vi "Read Plugin Data.vi"(8 "error in (no error)":errorcluster) -> (0 "error out":errorcluster, 2 "Queue Exists? Yes (T) No (F)":bool, 3 "Plugin Data":refnum<class "Generic Plugin.lvclass">)   [LabVIEW 2011, in "Generic Plugin.lvclass"]
uses:
  Generic Plugin.lvclass
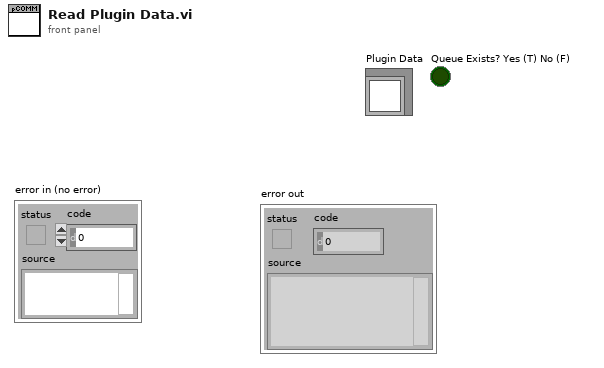
[diagram p1: front panel]
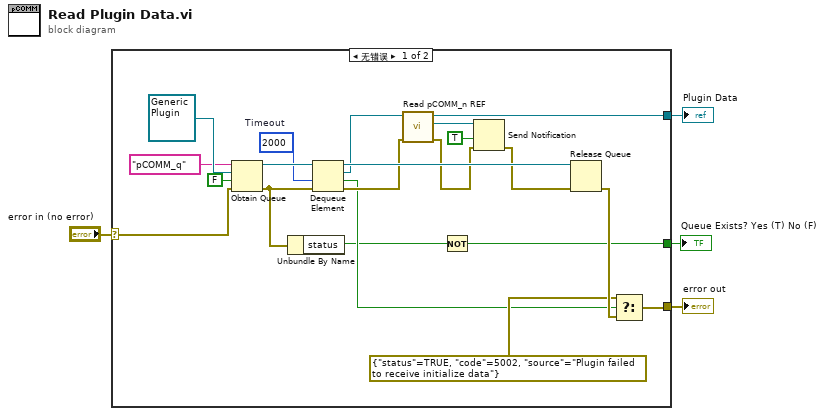
[diagram p0: block diagram]
diagram:
  n1 = case shown="无错误" "error in (no error)" {
    selector: "error in (no error)" -> [w23 w26]
    tunnel: [w18 w26] -> w4
    tunnel: [w14 _] -> w2
    tunnel: [w5 _] -> w1
    frame No Error {
      w21 = 2000  # Timeout
      n2 = Obtain Queue(name (unnamed)="pCOMM_q", element data type=refnum<class "Generic Plugin.lvclass"> refnum ("Generic Plugin.lvclass"), create if not found? (T)=FALSE, error in (no error)=w23) -> (queue out=w22:refnum<queue>, error out=w7:errorcluster)  [unwired: 1 in, 1 out]
      n3 = Unbundle By Name(w7) -> ("status"=w6:bool)
      n4 = Dequeue Element(queue=w22, timeout in ms (-1)=w21, error in (no error)=w7) -> (queue out=w17:refnum<queue>, element=w15:refnum<class "Generic Plugin.lvclass">, timed out?=w8:bool, error out=w11:errorcluster)
      n5 = call "Read pCOMM_n REF.vi"("error in (no error)"=w11, "Generic Plugin in"=w15) -> ("error out"=w10:errorcluster, "pCOMM_n REF"=w13:refnum<notifier>, "Generic Plugin out"=w14:refnum<class "Generic Plugin.lvclass">)  [unwired: 7 in]
      n6 = Not(x=w6) -> (.not. x?=w5:bool)
      n7 = Send Notification(notification=TRUE, notifier=w13, error in (no error)=w10) -> (error out=w12:errorcluster)  [unwired: 1 out]
      n8 = Release Queue(queue=w17, error in (no error)=w12) -> (error out=w20:errorcluster)  [unwired: 1 in, 2 out]
      n9 = Select(t=errorcluster {"status"=TRUE, "code"=5002, "source"="Plugin failed to receive initialize data"}, s=w8, f=w20) -> (s? t:f=w18:errorcluster)
    }
    frame Error {
    }
  }
  "error out" <- w4
  "Plugin Data" <- w2
  "Queue Exists? Yes (T) No (F)" <- w1
